vi "GetAttrib.vi"(8 "error in (no error)":errorcluster, 10 "Attrib":string, 11 "Refnum in":refnum<k20>) -> (0 "error out":errorcluster, 2 "Value":string, 3 "Refnum out":refnum<k20>)   [LabVIEW 2013]
uses:
  <resource>/objmgr/DOMUserDefRef.rc
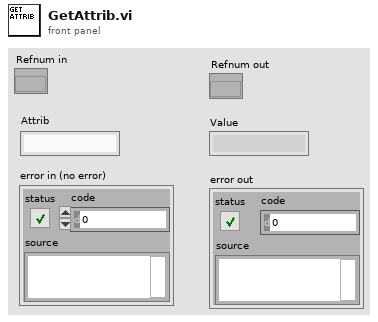
[diagram p1: front panel]
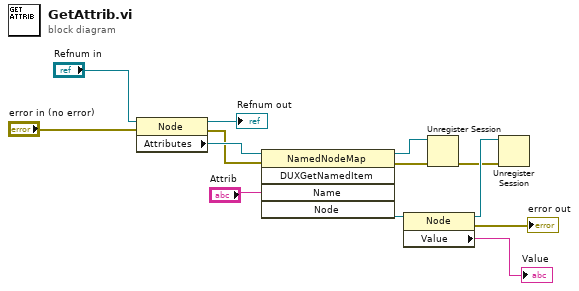
[diagram p0: block diagram]
diagram:
  n1 = property class="Node"(reference="Refnum in", error in="error in (no error)") -> (reference out=→"Refnum out":refnum<k20>, error out=w4:errorcluster, "Attributes"=w8:refnum<k20>)
  n2 = invoke class="NamedNodeMap" method="DUXGetNamedItem"(reference=w8, error in=w4, "Name"="Attrib") -> (reference out=w1:refnum<k20>, error out=w3:errorcluster, "Node"=w10:refnum<k20>)  [unwired: 2 in, 2 out]
  n3 = property class="Node"(reference=w10) -> (reference out=w12:refnum<k20>, error out=→"error out":errorcluster, "Value"=→"Value":string)  [unwired: 1 in]
  n4 = Unregister Session(8:w3, 11:w1) -> (0:w2:errorcluster)
  n5 = Unregister Session(8:w2, 11:w12) -> ()  [unwired: 1 out]
